vi "XY Graph Smoothen Plot Data.vi"(4 "Polynomial Order (S-G, 3)":i32=3, 5 "Smoothness (Cubic Spline)":dbl[](array[numeric]), 6 "Side Points (S-G, 6)":i32=6, 7 "Weight (Cubic Spline, S-G)":dbl[](array[numeric]) format="%#.6g", 8 "Error In":errorcluster, 9 "balance parameter (Cubic Spline, -1: auto)":dbl=-1.0, 10 "Smoothing Filter (Cubic Spline)":enum16{"None", "Cubic Spline", "Savitzky–Golay"}(ring)=enum."Cubic Spline", 11 "Plot":cluster{"X Array":dbl[], "Y Array":dbl[]}) -> (0 "error out":errorcluster, 3 "Cubic Splined Plot":cluster{"X Array":dbl[], "Y Array":dbl[]})   [LabVIEW 2021, in "XY Graph Add-Ons.lvlib"]
uses:
  <vilib>/Utility/error.llb/DialogType.ctl
  <vilib>/Analysis/3filter.llb/Savitzky-Golay Filter (DBL).vi
  XY Graph Add-Ons.lvlib
  <vilib>/Analysis/NI_AALPro.lvlib
  <vilib>/Analysis/NI_AALBase.lvlib
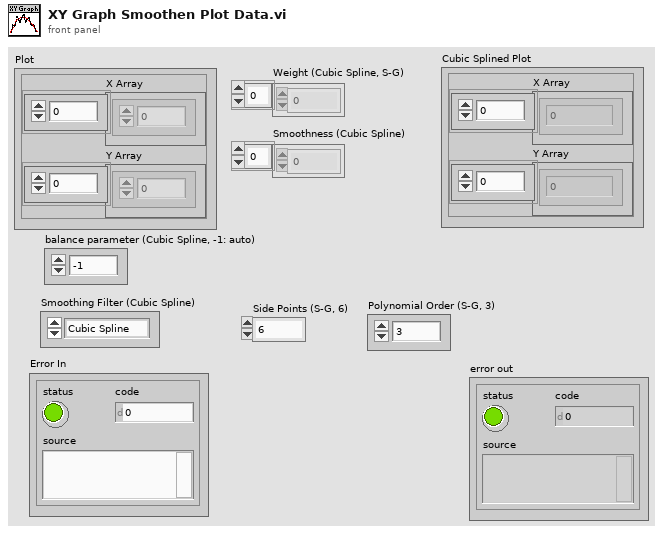
[diagram p1: front panel]
types:
  T1 = typedef "DialogType.ctl" = u16
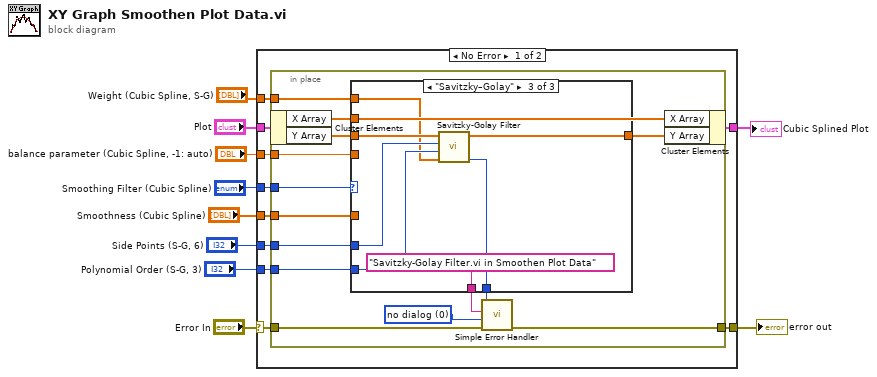
[diagram p0: block diagram]
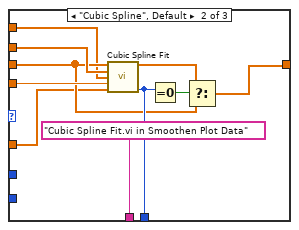
[diagram p3: hidden frame]
diagram:
  n1 = case shown="No Error" "Error In" {
    selector: "Error In" -> [w18 w53]
    tunnel: [w20 w53] -> w10
    tunnel: "balance parameter (Cubic Spline, -1: auto)" -> [w19 _]
    tunnel: "Plot" -> [w17 w54]
    tunnel: [w16 w54] -> w6
    tunnel: "Smoothing Filter (Cubic Spline)" -> [w15 _]
    tunnel: "Weight (Cubic Spline, S-G)" -> [w14 _]
    tunnel: "Smoothness (Cubic Spline)" -> [w13 _]
    tunnel: "Side Points (S-G, 6)" -> [w12 _]
    tunnel: "Polynomial Order (S-G, 3)" -> [w11 _]
    frame No Error {
      n2 = in-place {
        in-place-border: [w34] -> w20
        in-place-border: w19 -> [w31]
        in-place-border: w18 -> [w30]
        in-place-border: w15 -> [w25]
        in-place-border: w14 -> [w24]
        in-place-border: w13 -> [w23]
        in-place-border: w12 -> [w22]
        in-place-border: w11 -> [w21]
        w33 = T1 0 items=["no dialog", "OK message", "continue or stop message", "OK message + warnings", "continue/stop + warnings"] ("type of dialog (OK msg:1)")
        n3 = in-place-cluster #1(w17) -> ("X Array"=w29:dbl[], "Y Array"=w27:dbl[])
        n4 = case shown="\"Savitzky–Golay\"" w25 {
          tunnel: [_ "Cubic Spline Fit.vi in Smoothen Plot Data" ("error source (\" \")") "Savitzky-Golay Filter.vi in Smoothen Plot Data" ("error source (\" \")")] -> w32
          tunnel: w31 -> [_ w44 _]
          tunnel: w29 -> [_ w43 _]
          tunnel: [_ w42 w50] -> w28
          tunnel: w27 -> [w35 w40 w52]
          tunnel: [w35 w38 w51] -> w26
          tunnel: w24 -> [_ w37 w46]
          tunnel: w23 -> [_ w36 _]
          tunnel: w22 -> [_ _ w48]
          tunnel: w21 -> [_ _ w47]
          frame "None" {
          }
          frame "Cubic Spline", Default {
            n5 = call <vilib>:"Cubic Spline Fit.vi"("Y"=w40, "X"=w43, "Weight"=w37, "balance parameter"=w44, "Smoothness"=w36) -> ("Best Cubic Spline Fit"=w39:dbl[], "error"=w42:i32)  [unwired: 9 in]
            n6 = Equal To 0?(x=w42) -> (x = 0?=w41:bool)
            n7 = Select(t=w39, s=w41, f=w40) -> (s? t:f=w38:dbl[])
          }
          frame "Savitzky–Golay" {
            n8 = call-poly <vilib>:"Savitzky-Golay Filter.vi"("Weight"=w46, "polynomial order"=w47, "side points"=w48, "X"=w52) -> ("error"=w50:i32, "Filtered X"=w51:dbl[])  [unwired: 6 in]
          }
        }
        n9 = call <vilib>:"Simple Error Handler.vi"("error code (no error:0)"=w28, "error source (\" \")"=w32, "type of dialog (OK msg:1)"=w33, "error in (no error)"=w30) -> ("error out"=w34:errorcluster)  [unwired: 1 in, 4 out]
        n10 = in-place-cluster #1("X Array"=w29, "Y Array"=w26) -> (w16:cluster{"X Array":dbl[], "Y Array":dbl[]})
      }
    }
    frame Error {
    }
  }
  "error out" <- w10
  "Cubic Splined Plot" <- w6
